vi "Command handler.vi"(8 "error in (no error)":errorcluster, 11 "Cmd string (from UI)":string="test fieldscan_up.txt") -> (0 "error out":errorcluster)   [LabVIEW 2019]
uses:
  Controls/Log destination selector.ctl
  Controls/Test-run selector.ctl
  _Global variables 1.vi
panel:
  out "Arguments":string[](array[string])=["test", "fieldscan_up.txt"]
  # "Ex:\ntest <batch>\nrun <batch>\nor any device command"
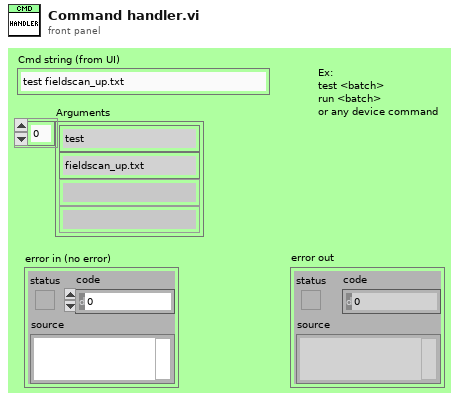
[diagram p1: front panel]
types:
  T1 = typedef "Log destination selector.ctl" = enum16{"UI", "File", "UI+file"}
  T2 = typedef "Test-run selector.ctl" = enum16{"Test", "Run"}
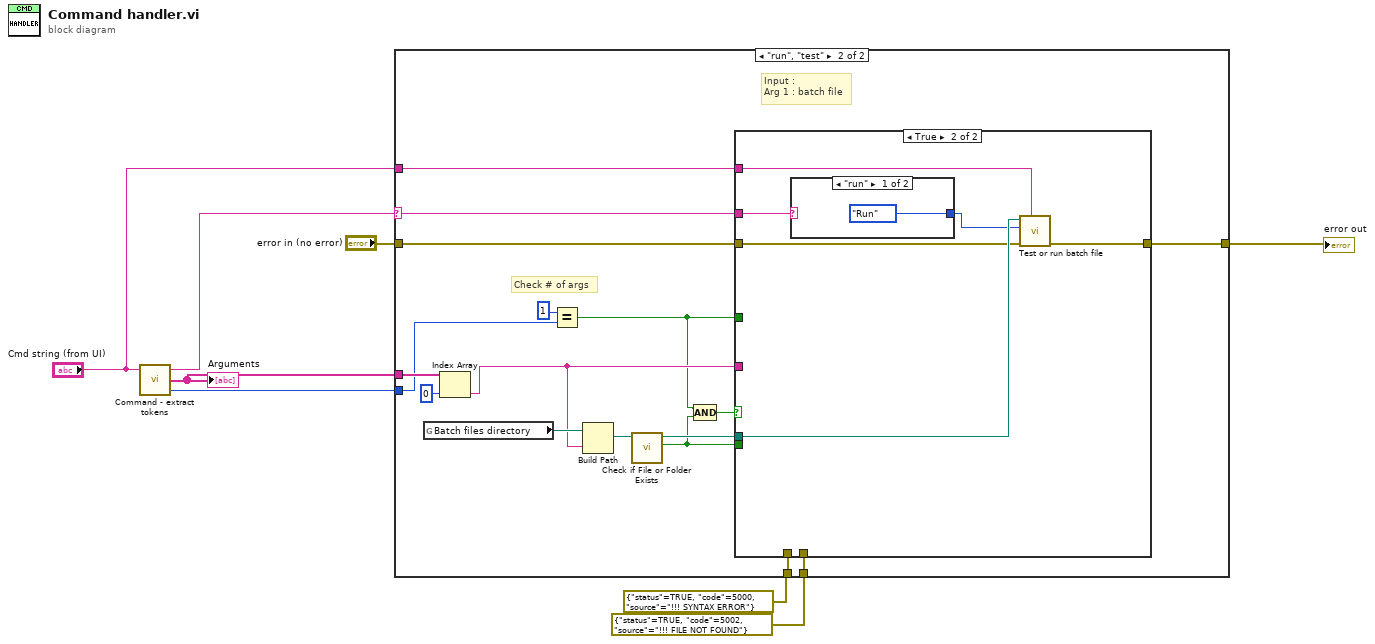
[diagram p0: block diagram]
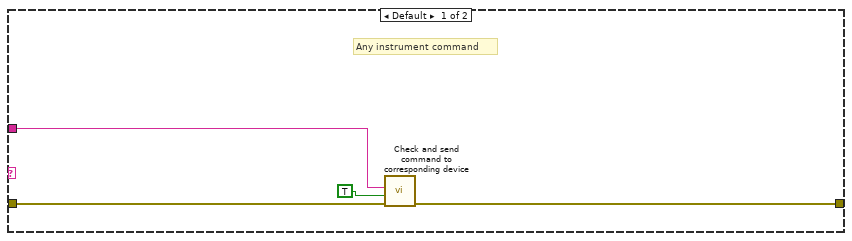
[diagram p2: hidden frame]
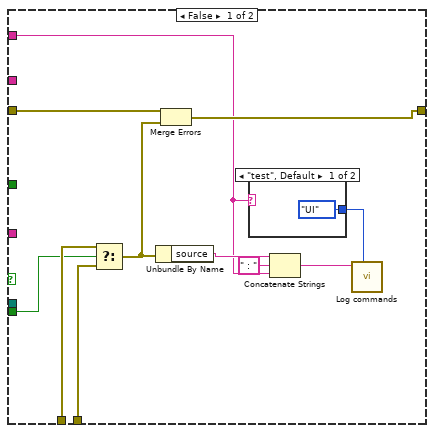
[diagram p3: hidden frame]
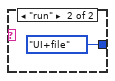
[diagram p4: hidden frame]
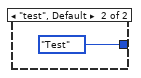
[diagram p5: hidden frame]
diagram:
  n1 = call "Command - extract tokens.vi"("Cmd string"="Cmd string (from UI)") -> ("N arg"=w4:u8, "Arguments"=w6:string[], "Command"=w5:string)  [unwired: 2 in]
  "Arguments" <- w6
  n2 = case shown="\"run\", \"test\"" w5 {
    selector: w5 -> [_ w13]
    tunnel: w6 -> [_ w28]
    tunnel: "error in (no error)" -> [w11 w25]
    tunnel: [w10 w24] -> w7
    tunnel: "Cmd string (from UI)" -> [w12 w23]
    tunnel: w4 -> [_ w18]
    tunnel: errorcluster {"status"=TRUE, "code"=5000, "source"="!!! SYNTAX ERROR"} ("error out") -> [_ w17]
    tunnel: errorcluster {"status"=TRUE, "code"=5002, "source"="!!! FILE NOT FOUND"} ("error out") -> [_ w16]
    frame Default {
      # "Any instrument command"
      n3 = call "Check and send command to corresponding device.vi"("error in (no error)"=w11, "Execute cmd (F)"=TRUE ("Log cmd to file (T)"), "Cmd string"=w12) -> ("error out"=w10:errorcluster)  [unwired: 7 in, 1 out]
    }
    frame "run", "test" {
      # "Check # of args"
      # "Input :\nArg 1 : batch file"
      n4 = global read "_Global variables 1.vi" "Batch files directory"() -> (w22:path)
      n5 = Index Array(array=w28, index=0) -> (element=w21:string)
      n6 = Equal?(x=1 ("y"), y=w18) -> (x = y?=w15:bool)
      n7 = Build Path(base path=w22, name or relative path=w21) -> (appended path=w20:path)
      n8 = call <vilib>:"Check if File or Folder Exists.vi"("path"=w20) -> ("file or folder exists?"=w14:bool, "dup path"=w19:path)  [unwired: 8 in, 1 out]
      n9 = Compound Arithmetic op=AND(w15, w14) -> (w27:bool)
      n10 = case shown="True" w27 {
        tunnel: w21 -> [_ _]
        tunnel: w25 -> [w40 w47]
        tunnel: [w39 w46] -> w24
        tunnel: w23 -> [w31 w45]
        tunnel: w19 -> [_ w48]
        tunnel: w17 -> [w38 _]
        tunnel: w16 -> [w37 _]
        tunnel: w15 -> [_ _]
        tunnel: w14 -> [w36 _]
        tunnel: w13 -> [_ w44]
        frame False {
          n11 = Select(t=w38, s=w36, f=w37) -> (s? t:f=w35:errorcluster)
          n12 = Unbundle By Name(w35) -> ("source"=w33:string)
          n13 = Merge Errors(w40, w35) -> (w39:errorcluster)
          n14 = case shown="\"test\", Default" w31 {
            tunnel: [Log_destination_selector."UI" ("Log destination") Log_destination_selector."UI+file" ("Log destination")] -> w30
            frame "test", Default {
            }
            frame "run" {
            }
          }
          n15 = Concatenate Strings(w33, " : " ("string"), w31) -> (w32:string)
          n16 = call "Log commands.vi"("Log destination"=w30, "text to log"=w32) -> ()  [unwired: 9 in, 1 out]
        }
        frame True {
          n17 = case shown="\"run\"" w44 {
            tunnel: [Test-run_selector."Run" ("Action") Test-run_selector."Test" ("Action")] -> w43
            frame "run" {
            }
            frame "test", Default {
            }
          }
          n18 = call "Test or run batch file.vi"("Cmd string (to log)"=w45, "error in"=w47, "Action"=w43, "Batch file path"=w48) -> ("error out"=w46:errorcluster)  [unwired: 6 in, 1 out]
        }
      }
    }
  }
  "error out" <- w7
